vi "Init_Test.vi"(8 "error in (no error)":errorcluster caption="entrée d'erreur (pas d'erreur)", 11 "Flash_Jlink en entrée":refnum<class "Flash_AVRDUDE.lvclass">) -> (0 "error out":errorcluster caption="sortie d'erreur", 3 "Flash_Jlink en sortie":refnum<class "Flash_AVRDUDE.lvclass">)   [LabVIEW 2020, in "Library Test.lvlib" / "Flash_AVRDUDE.lvclass"]
uses:
  Flash_AVRDUDE.lvclass
  C:/Users/ngarcin/OneDrive - Altyor/Standard TB/Class/Test/Test (Default)/Test (Default).lvclass
  Commun VI/TypeDef/Commande Test/Commande Type Test.ctl
  Commun VI/TypeDef/Commande Test/Commande Value Type.ctl
  Test_Without_Instr/Test_Without_Inst.lvclass
  Flash_AVRDUDE.lvclass/Flash_AVRDUDE.ctl
  Commun VI/Library Commun.lvlib
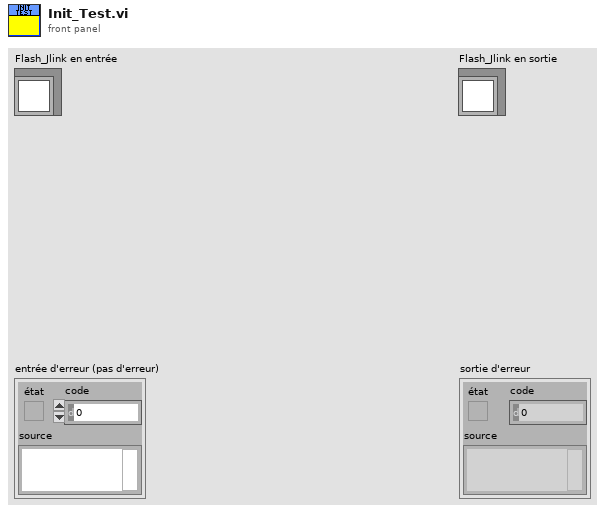
[diagram p1: front panel]
types:
  T1 = typedef "Library Commun.lvlib/Commande Value Type.ctl" = enum16{"None", "String", "Number", "Timestamp", "Boolean", "Array"}
  T2 = typedef "Library Commun.lvlib/Commande Type Test.ctl" = enum16{"Function", "Test", "Calculation"}
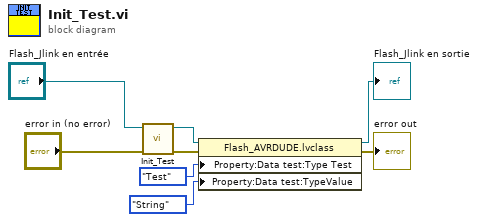
[diagram p0: block diagram]
diagram:
  n1 = call-parent "Init_Test.vi"("error in (no error)"="error in (no error)", "Test_Without_Inst en entrée"="Flash_Jlink en entrée") -> ("error out"=w1:errorcluster, "Test_Without_Inst en sortie"=w2:refnum<class "Flash_AVRDUDE.lvclass">)  [unwired: 8 in]
  n2 = property class="Flash_AVRDUDE.lvclass"(reference=w2, error in=w1, "Property:Data test:Type Test"=Commande_Type_Test."Test" ("Type Test"), "Property:Data test:TypeValue"=Commande_Value_Type."String" ("TypeValue")) -> (reference out=→"Flash_Jlink en sortie":refnum<class "Flash_AVRDUDE.lvclass">, error out=→"error out":errorcluster)
